vi "EnFlo_Coordinate_transforms.vi"(3 "Input":dbl[](array[numeric])=[0.0, 0.0, 0.0] format="%.2f", 5 "Mode":enum16{"XYZ to Channel", "Channel to XYZ"}(ring)) -> (0 "Output":dbl[](array[numeric]) format="%.2f", 1 "Z theta":dbl format="%.2f", 2 "X theta":dbl format="%.2f")   [LabVIEW 2010]
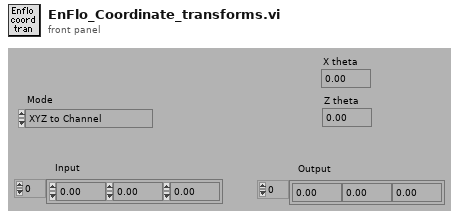
[diagram p1: front panel]
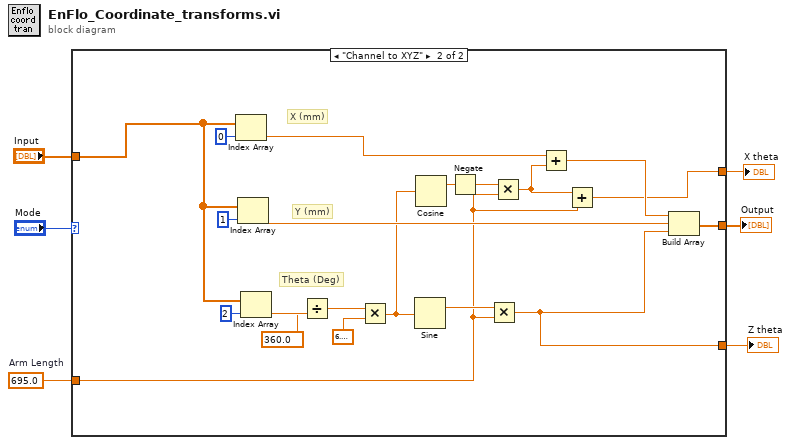
[diagram p0: block diagram]
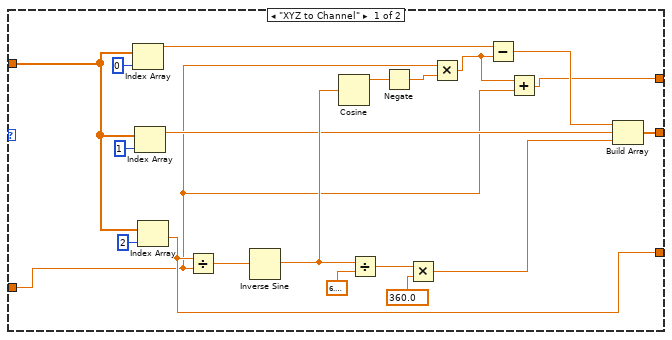
[diagram p2: hidden frame]
diagram:
  w3 = 695.0  # Arm Length
  n1 = case shown="\"Channel to XYZ\"" "Mode" {
    tunnel: "Input" -> [w23 w46]
    tunnel: [w18 w42] -> w4
    tunnel: w3 -> [w8 w28]
    tunnel: [w7 w27] -> w2
    tunnel: [w11 w31] -> w1
    frame "XYZ to Channel" {
      n2 = Index Array(array=w23, index=0 ("Index")) -> (element=w14:dbl)
      n3 = Index Array(array=w23, index=1 ("Index")) -> (element=w12:dbl)
      n4 = Index Array(array=w23, index=2 ("Index")) -> (element=w11:dbl)
      n5 = Divide(x=w11, y=w8) -> (x/y=w22:dbl)
      n6 = Inverse Sine(1:w22) -> (0:w15:dbl)
      n7 = Cosine(x=w15) -> (cos(x)=w17:dbl)
      n8 = Divide(x=w15, y=6.283185307179586) -> (x/y=w21:dbl)
      n9 = Negate(x=w17) -> (-x=w10:dbl)
      n10 = Multiply(x=w21, y=360.0) -> (x*y=w16:dbl)
      n11 = Multiply(x=w8, y=w10) -> (x*y=w9:dbl)
      n12 = Subtract(x=w14, y=w9) -> (x-y=w13:dbl)
      n13 = Add(x=w9, y=w8) -> (x+y=w7:dbl)
      n14 = Build Array(w13, w12, w16) -> (w18:dbl[])
    }
    frame "Channel to XYZ" {
      # "Theta (Deg)"
      # "Y (mm)"
      # "X (mm)"
      n15 = Index Array(array=w46, index=0 ("Index")) -> (element=w40:dbl)
      n16 = Index Array(array=w46, index=1 ("Index")) -> (element=w41:dbl)
      n17 = Index Array(array=w46, index=2 ("Index")) -> (element=w38:dbl)
      n18 = Divide(x=w38, y=360.0) -> (x/y=w36:dbl)
      n19 = Multiply(x=w36, y=6.283185307179586) -> (x*y=w34:dbl)
      n20 = Sine(x=w34) -> (sin(x)=w32:dbl)
      n21 = Cosine(x=w34) -> (cos(x)=w33:dbl)
      n22 = Negate(x=w33) -> (-x=w30:dbl)
      n23 = Multiply(x=w32, y=w28) -> (x*y=w31:dbl)
      n24 = Multiply(x=w30, y=w28) -> (x*y=w29:dbl)
      n25 = Add(x=w40, y=w29) -> (x+y=w39:dbl)
      n26 = Add(x=w29, y=w28) -> (x+y=w27:dbl)
      n27 = Build Array(w39, w41, w31) -> (w42:dbl[])
    }
  }
  "Output" <- w4
  "X theta" <- w2
  "Z theta" <- w1
